vi "正逆解测试.vi"() -> ()   [LabVIEW 2014]
panel:
  out "误差2":dbl[](array[numeric])
  out "验证输出2":dbl[](array[numeric])=[-2177.0, -1.4612052517330483e-10, 558.0000000005964, 1.0] format="%#.6f"
  out "运动学逆解2":dbl[](array[numeric])
  out "误差":dbl[](array[numeric])
  out "逆运动学输出":dbl[](array[numeric])=[0.0, 0.0, 0.0, 0.0, 4.859887553275934e-12, 0.0] format="%#.3f"
  out "正解输出":dbl[](array[numeric])=[0.19999999999996898, -1.0341155355512858e-14, 0.3000000000000207] format="%#.6f"
  out "验证输出":dbl[](array[numeric])=[0.19999999999996898, -1.0341155355512858e-14, 0.3000000000000207] format="%#.6f"
  in  "关节数":dbl=6.0
  in  "正运动学输入":dbl[](array[numeric])=[0.0, 0.0, 0.0, 0.0, 0.0, 0.0]
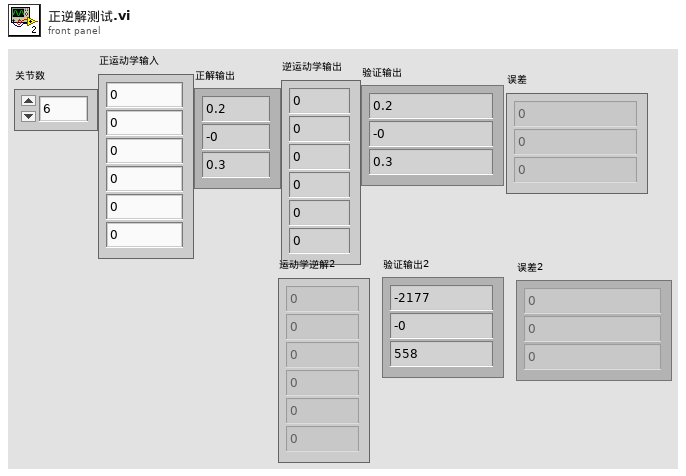
[diagram p1: front panel]
types:
  T1 = typedef "Real Matrix NI_Silver.ctl" = dbl[][]
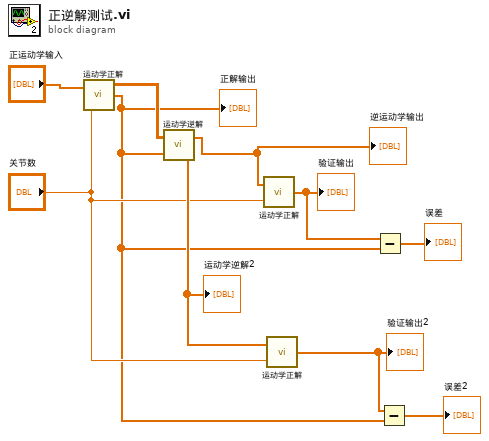
[diagram p0: block diagram]
diagram:
  n1 = call "运动学正解.vi"("正运动学输入"="正运动学输入", "关节数"="关节数") -> ("Tx"=w9:T1, "正解输出"=w2:dbl[])  [unwired: 1 out]
  "正解输出" <- w2
  n2 = call "运动学逆解.vi"("逆运动学输入"=w2, "机械臂末端姿态"=w9) -> ("运动学逆解2"=w5:dbl[], "运动学逆解1"=w6:dbl[])
  "逆运动学输出" <- w6
  "运动学逆解2" <- w5
  n3 = call "运动学正解.vi"("正运动学输入"=w6, "关节数"="关节数") -> ("正解输出"=w8:dbl[])  [unwired: 2 out]
  "验证输出" <- w8
  n4 = call "运动学正解.vi"("正运动学输入"=w5, "关节数"="关节数") -> ("正解输出"=w3:dbl[])  [unwired: 2 out]
  "验证输出2" <- w3
  n5 = Subtract(x=w8, y=w2) -> (x-y=→"误差":dbl[])
  n6 = Subtract(x=w3, y=w2) -> (x-y=→"误差2":dbl[])
